vi "TDS_ConfigureChannel.vi"(7 "instrument handle":refnum<k15>, 8 "error in":errorcluster, 11 "VI ServerCluster":T1) -> (0 "error out":errorcluster)   [LabVIEW 2020]
uses:
  LabVIEW 2020 Toolkits/VI Server Toolkit/VI Server_TypeDefs/VI Server_RefsCluster.ctl
  LabVIEW 2020 Toolkits/VI Server Toolkit/VI Server Libraries/VI Server_GetControl.llb/VI Server_STR_Get.vi
  LabVIEW 2020 Toolkits/VI Server Toolkit/VI Server Libraries/VI Server_GetControl.llb/VI Server_Bool_Get.vi
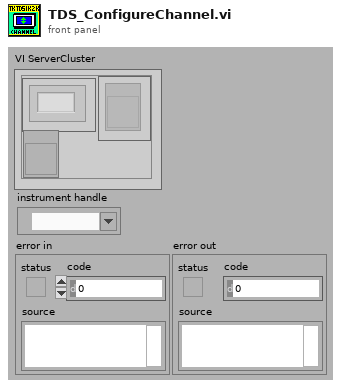
[diagram p1: front panel]
types:
  T1 = typedef "VI Server_RefsCluster.ctl" = cluster{"Labels":string[], "Refs":refnum<vi>[], "VI Ref":refnum<vi>}
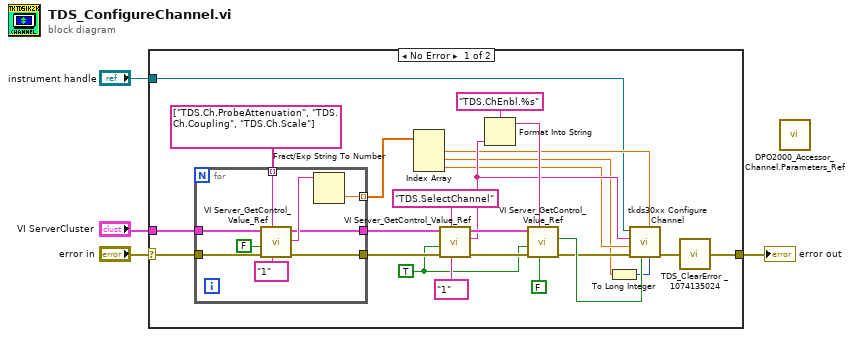
[diagram p0: block diagram]
diagram:
  n1 = case shown="No Error" "error in" {
    selector: "error in" -> [w8 w38]
    tunnel: "VI ServerCluster" -> [w11 _]
    tunnel: "instrument handle" -> [w9 _]
    tunnel: [w6 w38] -> w3
    frame No Error {
      w5 = TRUE ("SingleInstance")
      n2 = for {
        tunnel: string[] ["TDS.Ch.ProbeAttenuation", "TDS.Ch.Coupling", "TDS.Ch.Scale"] -> [w36] mode=indexing
        tunnel: [w34] -> w12 mode=indexing
        tunnel: w11 -> [w31]
        tunnel: [w30] -> w19
        tunnel: w8 -> [w33]
        tunnel: [w32] -> w16
        n3 = call-poly "VI Server_GetControl_Value_Ref.vi"("DataType"="1" ("TDS.Ch.ProbeAttenuation 2"), "Control.Label"=w36, "error in"=w33, "SingleInstance"=FALSE, "VI Server.RefsCluster"=w31) -> ("error out"=w32:errorcluster, "Value"=w35:string, "VI Server.RefsCluster.DUP"=w30:T1)  [unwired: 3 in, 1 out]
        n4 = Fract/Exp String To Number(string=w35) -> (number=w34:dbl)  [unwired: 3 in, 1 out]
      }
      n5 = Index Array(array=w12) -> (element #1=w13:dbl, element #2=w14:dbl, element #3=w20:dbl)  [unwired: 3 in]
      n6 = call-poly "VI Server_GetControl_Value_Ref.vi"("DataType"="1" ("TDS.Ch.ProbeAttenuation 2"), "Control.Label"="TDS.SelectChannel" ("Label"), "error in"=w16, "SingleInstance"=w5, "VI Server.RefsCluster"=w19) -> ("error out"=w23:errorcluster, "Value"=w22:string, "VI Server.RefsCluster.DUP"=w25:T1)  [unwired: 3 in, 1 out]
      n7 = Format Into String(format string="TDS.ChEnbl.%s", w22) -> (resulting string=w26:string)  [unwired: 2 in, 1 out]
      n8 = call-poly "VI Server_GetControl_Value_Ref.vi"("DataType"=FALSE, "Control.Label"=w26, "error in"=w23, "SingleInstance"=w5, "VI Server.RefsCluster"=w25) -> ("error out"=w24:errorcluster, "Value"=w28:bool)  [unwired: 3 in, 2 out]
      n9 = To Long Integer(number=w14) -> (32bit integer=w15:i32)
      n10 = call "tkds30xx Configure Channel.vi"("Vertical Offset (0)"=w13, "Vertical Coupling (DC)"=w15, "Channel Enabled (True)"=w28, "error in (no error)"=w24, "Probe Attenuation (1.0)"=w20, "Channel Name (Channel 1)"=w22, "instrument handle"=w9) -> ("error out"=w7:errorcluster)  [unwired: 3 in, 1 out]
      n11 = call "TDS_ClearError _1074135024.vi"("error in"=w7) -> ("error out"=w6:errorcluster)  [unwired: 4 in]
    }
    frame Error {
    }
  }
  "error out" <- w3
  n12 = call "DPO2000_Accessor_Channel.Parameters_Ref.vi"() -> ()  [unwired: 6 in, 1 out]
